vi "Register ValueChanged Callback.vi"(8 "error in":errorcluster, 10 "onValueChanged":refnum<user-event>, 11 "Custom Events in":refnum<class "Custom Events.lvclass">) -> (0 "error out":errorcluster, 2 "Event Callback Refnum":refnum<k27>, 3 "Custom Events out":refnum<class "Custom Events.lvclass">)   [LabVIEW 2024, in "SourceGrid.lvlib" / "Custom Events.lvclass"]
uses:
  Custom Events.lvclass
  Cells/Cell Context/Cell Context.lvclass
  Custom Events.lvclass/Custom Events.ctl
  ValueChanged Callback.vi
  D:/git/Sourcegrid-LabVIEW/dll/SourceGrid.dll
  dll/SourceGrid.dll
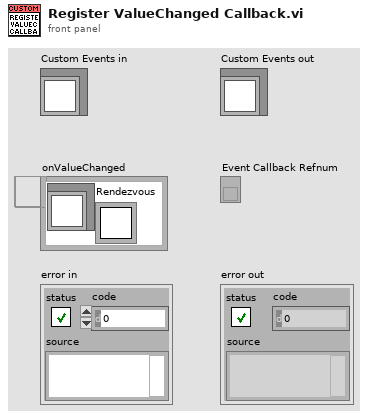
[diagram p1: front panel]
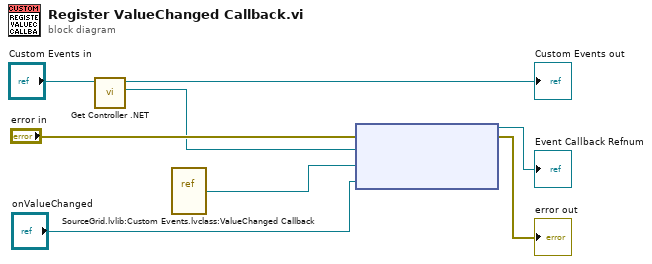
[diagram p0: block diagram]
diagram:
  n1 = call "Get Controller .NET.vi"("Custom Events in"="Custom Events in") -> ("CustomEvents .NET"=w5:refnum<k24>)  [unwired: 9 in, 1 out]
  n2 = vi-ref "SourceGrid.lvlib:Custom Events.lvclass:ValueChanged Callback.vi"() -> (w1:refnum<vi>)
  n3 = node("error in", w5, w1, "onValueChanged") -> (→"Event Callback Refnum":refnum<k27>, →"error out":errorcluster)  [unwired: 1 in]
  "Custom Events out" <- "Custom Events in"
